vi "GetMethods.vi"(8 "error in (no error)":errorcluster, 11 "UMLClass in":refnum<class "UMLClass.lvclass">) -> (0 "error out":errorcluster, 2 "Methods":string[](array[string])=["Draw ()", "Scale ()", "Move ()"], 3 "UMLClass out":refnum<class "UMLClass.lvclass">)   [LabVIEW 2021, in "Picture2D.lvlib" / "UMLClass.lvclass"]
uses:
  UMLClass.lvclass
  UMLClass.lvclass/UMLClass.ctl
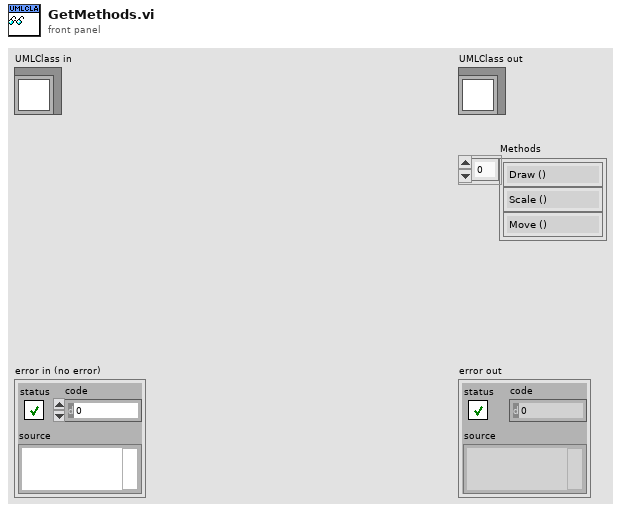
[diagram p1: front panel]
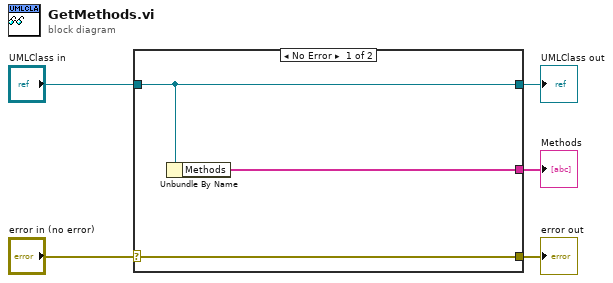
[diagram p0: block diagram]
diagram:
  n1 = case shown="No Error" "error in (no error)" {
    selector: "error in (no error)" -> [w8 w9]
    tunnel: [w8 w9] -> w4
    tunnel: [w7 w10] -> w2
    tunnel: "UMLClass in" -> [w7 w10]
    tunnel: [w6 _] -> w1
    frame No Error {
      n2 = Unbundle By Name(w7) -> ("Methods"=w6:string[])
    }
    frame Error {
    }
  }
  "error out" <- w4
  "UMLClass out" <- w2
  "Methods" <- w1
